vi "Post Result.vi"(8 "error in (no error)":errorcluster, 11 "DBL Result Class in":refnum<class "DBL Result Class.lvclass">) -> (0 "error out":errorcluster, 3 "DBL Result Class out":refnum<class "DBL Result Class.lvclass">)   [LabVIEW 2018, in "DBL Result Class.lvclass"]
uses:
  DBL Result Class.lvclass
  DBL Result Class.lvclass/DBL Result Class.ctl
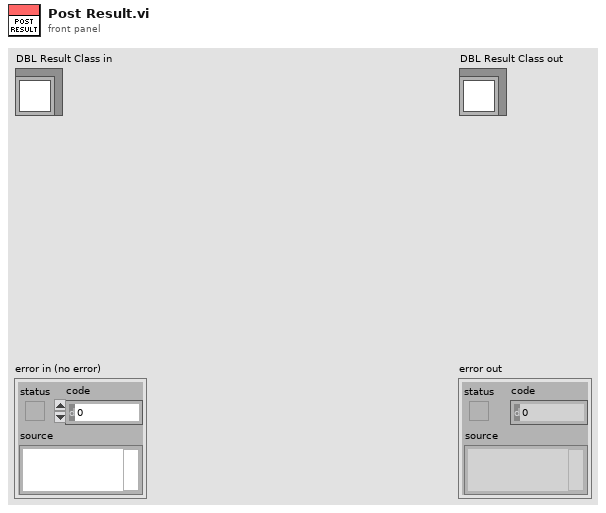
[diagram p1: front panel]
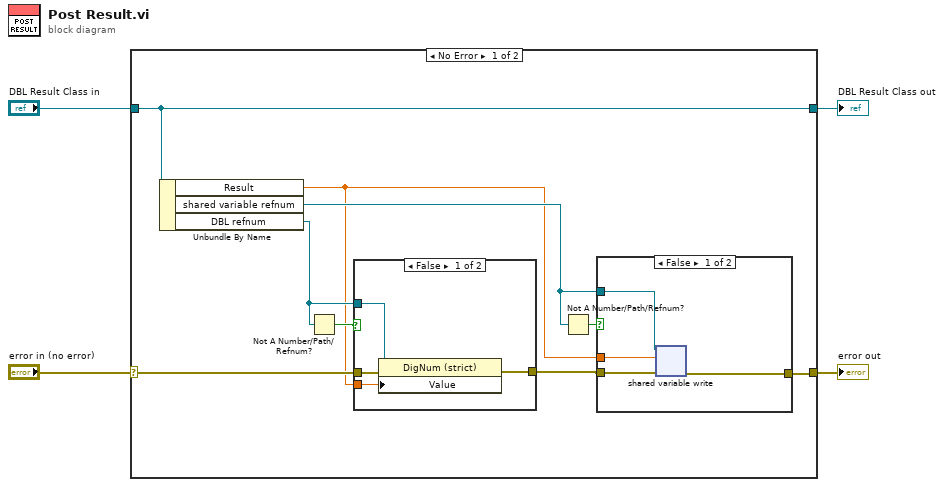
[diagram p0: block diagram]
diagram:
  n1 = case shown="No Error" "error in (no error)" {
    selector: "error in (no error)" -> [w8 w25]
    tunnel: [w6 w25] -> w3
    tunnel: [w13 w24] -> w1
    tunnel: "DBL Result Class in" -> [w13 w24]
    frame No Error {
      n2 = Unbundle By Name(w13) -> ("Result"=w5:dbl, "shared variable refnum"=w9:refnum<k21>, "DBL refnum"=w10:refnum<vi>)
      n3 = Not A Number/Path/Refnum?(number/path/refnum=w10) -> (NaN/Path/Refnum?=w11:bool)
      n4 = case shown="False" w11 {
        tunnel: w10 -> [w17 _]
        tunnel: w8 -> [w16 w18]
        tunnel: [w15 w18] -> w7
        tunnel: w5 -> [w14 _]
        frame False {
          n5 = property class="DigNum (strict)"(reference=w17, error in=w16, "Value"=w14) -> (error out=w15:errorcluster)  [unwired: 1 out]
        }
        frame True {
        }
      }
      n6 = Not A Number/Path/Refnum?(number/path/refnum=w9) -> (NaN/Path/Refnum?=w12:bool)
      n7 = case shown="False" w12 {
        tunnel: w7 -> [w22 w23]
        tunnel: w9 -> [w21 _]
        tunnel: [w20 w23] -> w6
        tunnel: w5 -> [w19 _]
        frame False {
          n8 = shared-variable-write(w21, w22, w19) -> (w20:errorcluster)  [unwired: 1 out]
        }
        frame True {
        }
      }
    }
    frame Error {
    }
  }
  "error out" <- w3
  "DBL Result Class out" <- w1
